vi "find_patches_test.vi"() -> ()   [LabVIEW 2017]
uses:
  gVision/gVision.lvlib
  <vilib>/vision/NI_Vision_Development_Module.lvlib
panel:
  out "Patches":T1(array[cluster]) {"x" format="%#_3g"; "y" format="%#_3g"; "aspect ratio" format="%#_3g"; "size" format="%#_3g"; "image-x" format="%#_3g"; "image-y" format="%#_3g"}
  out "Number of Fiducials":i32
  in  "Fiducial Parameters":T2={"dilateSize"=5, "sizeMin"=0.0, "sizeMax"=10.0, "aspectRatioMin"=0.9, "aspectRatioMax"=1.1, "colorGroups"=2, "fieldOfViewX"=1.4, "fieldOfViewY"=1.048}
  in  "File Path":path=path "C:/Users/cfang/Desktop/pixel-gantry-control/Data/HDI_fid.png"
  out "error out":errorcluster
  out "Image":T3(plugin-control)
  in  "debug":bool
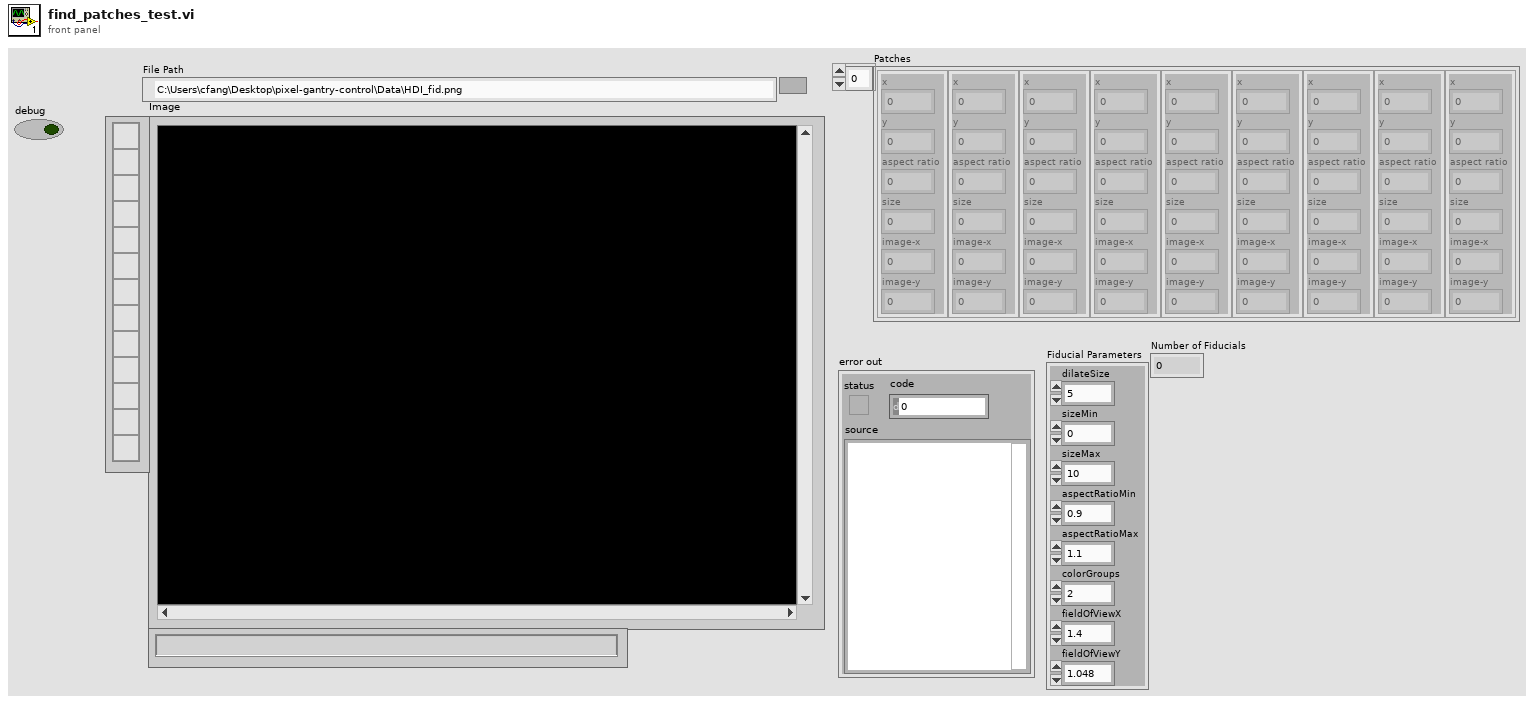
[diagram p1: front panel]
types:
  T1 = cluster{"x":dbl, "y":dbl, "aspect ratio":dbl, "size":dbl, "image-x":dbl, "image-y":dbl}[]
  T2 = cluster{"dilateSize":i32, "sizeMin":sgl, "sizeMax":sgl, "aspectRatioMin":sgl, "aspectRatioMax":sgl, "colorGroups":i32, "fieldOfViewX":sgl, "fieldOfViewY":sgl}
  T3 = typedef "IMAQ Image.ctl" = refnum<image>
  T4 = typedef "Image Type" = u32
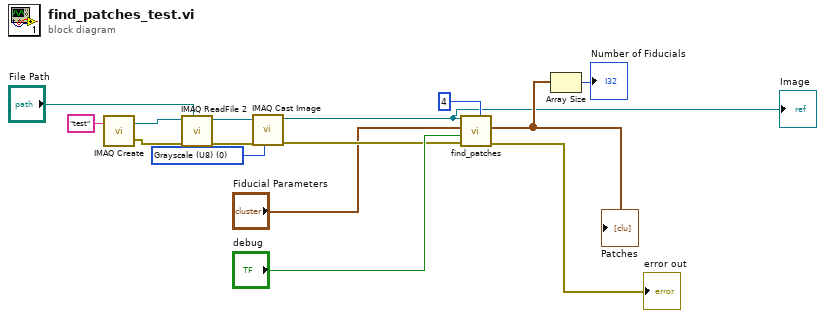
[diagram p0: block diagram]
diagram:
  w6 = T4 0 items=["Grayscale (U8)", "Grayscale (I16)", "Grayscale (SGL)", "Complex (CSG)", "RGB (U32)", "HSL (U32)", "RGB (U64)", "Grayscale (U16)"] ("Image Type")
  n1 = call "IMAQ Create"("Image Name"="test") -> ("New Image"=w14:T3, "error out"=w12:errorcluster)  [unwired: 4 in]
  n2 = call "IMAQ ReadFile 2"("File Path"="File Path", "error in (no error)"=w12, "Image"=w14) -> ("error out"=w9:errorcluster, "Image Out"=w7:T3)  [unwired: 4 in, 3 out]
  n3 = call "IMAQ Cast Image"("Image Type"=w6, "error in (no error)"=w9, "Image Src"=w7) -> ("error out"=w8:errorcluster, "Image Dst Out"=w1:T3)  [unwired: 7 in]
  "Image" <- w1
  n4 = call "find_patches.vi"("Shrink Factor"=4, "error in"=w8, "debug"="debug", "Fiducial Parameters"="Fiducial Parameters", "Image"=w1) -> ("error out"=→"error out":errorcluster, "Patches"=w2:T1)  [unwired: 5 in]
  "Patches" <- w2
  n5 = Array Size(array=w2) -> (size(s)=→"Number of Fiducials":i32)
